vi "boonton_main.vi"() -> ()   [LabVIEW 2011]
uses:
  delay_time.vi
panel:
  out "Bias":string
  out "Loop Time 2":dbl
  in  "Sample Time":dbl
  out "Loop Time":dbl
  out "loop cnt":dbl
  in  "Destination File 2":path
  in  "Delay time":dbl
  in  "Destination File":path
  out "Command Read error out":errorcluster
  in  "Command File":path
  out "Result":string
  out "VISA error out":errorcluster
  in  "error in (no error)":errorcluster
  out "VISA Out":refnum<visa-resource-name>
  in  "VISA In":refnum<visa-resource-name>
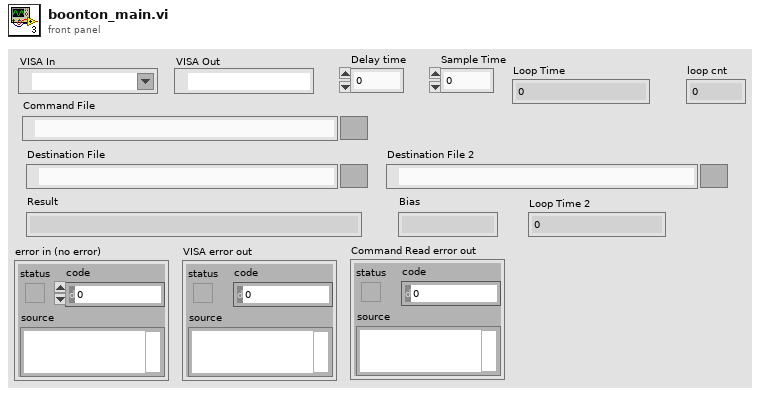
[diagram p1: front panel]
types:
  T1 = enum16{"open", "replace", "create", "open or create", "replace or create", "replace or create with confirmation"}
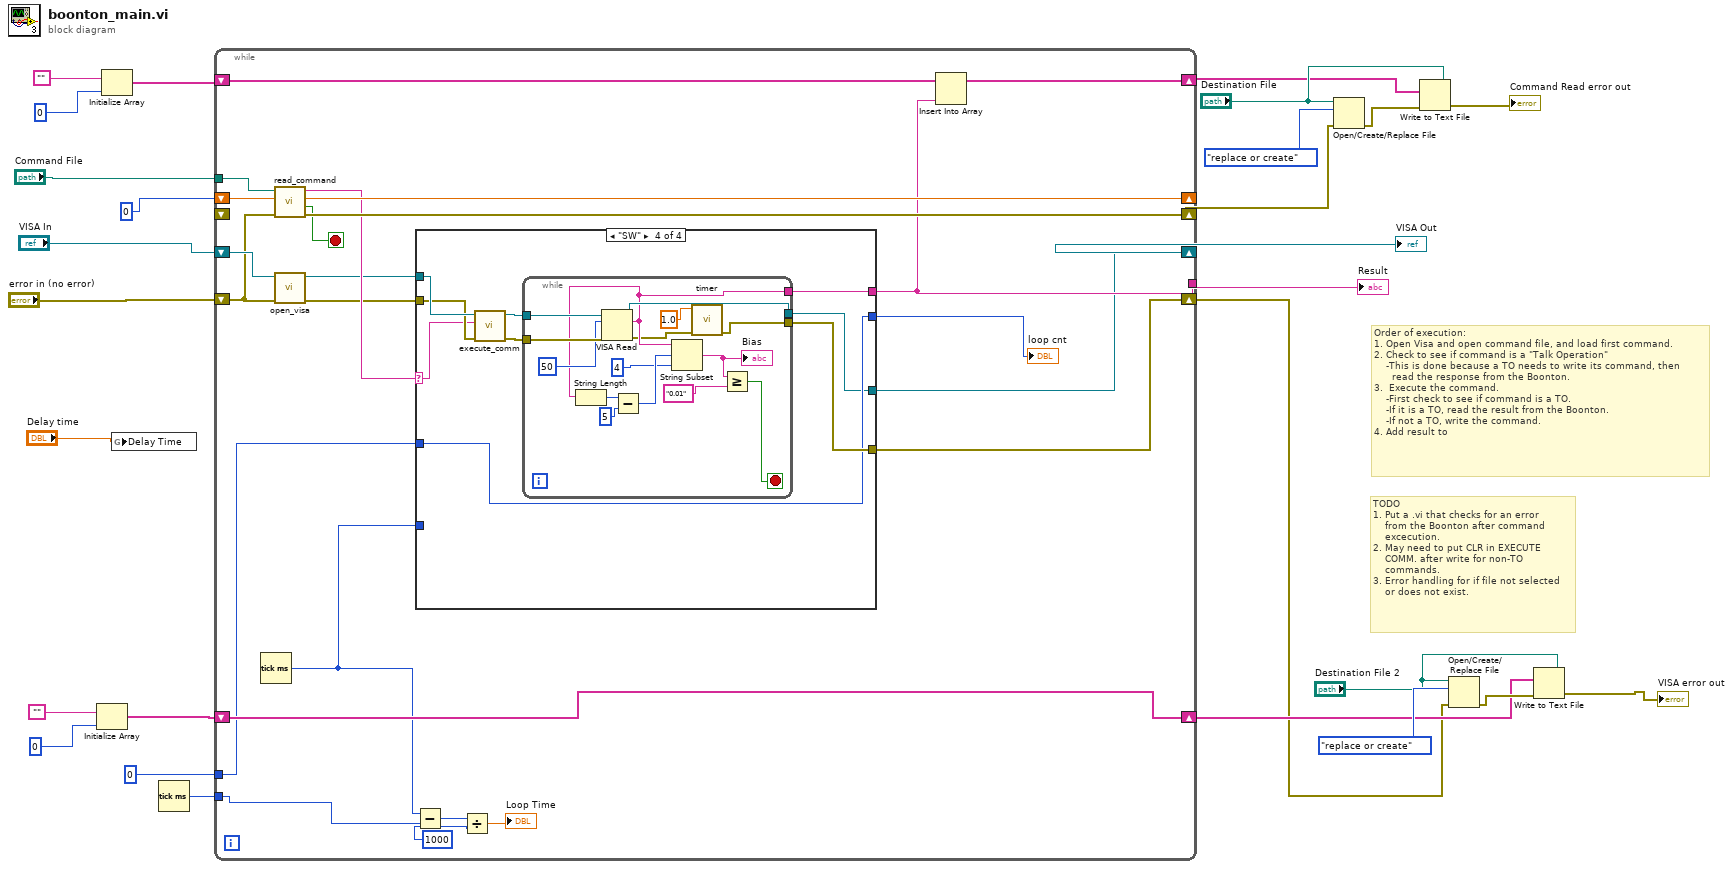
[diagram p0: block diagram]
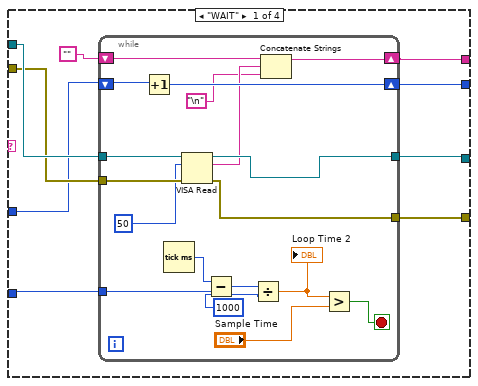
[diagram p2: hidden frame]
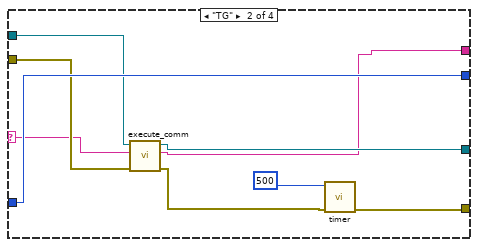
[diagram p3: hidden frame]
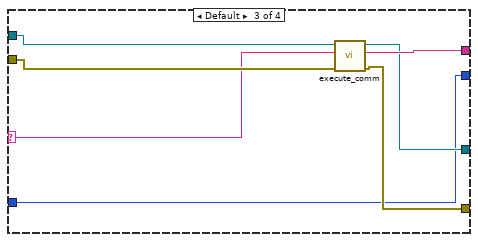
[diagram p4: hidden frame]
diagram:
  # "TODO\n1. Put a .vi that checks for an error\n    from the Boonton after command\n    excecution.\n2. May need to put CLR in EXECUTE\n    COMM. after write for non-TO\n    commands.\n3. Error handling for if file not selected\n    or does not exist."
  # "Order of execution:\n1. Open Visa and open command file, and load first command.\n2. Check to see if command is a \"Talk Operation\"\n    -This is done because a TO needs to write its command, then\n      read the response from the Boonton.\n3.  Execute the command.\n    -First check to see if command is a TO.\n    -If it is a TO, read the result from the Boonton.\n    -If not a TO, write the command.\n4. Add result to"
  n1 = Initialize Array("", 0) -> (w10:string[])
  n2 = Initialize Array("", 0) -> (w19:string[])
  n3 = global write "delay_time.vi" "Delay Time"("Delay time") -> ()
  n4 = Tick Count (ms)() -> (millisecond timer value=w3:u32)
  n5 = while {
    tunnel: [w36] -> w25
    tunnel: "Command File" -> [w47]
    shift-right: [w34] -> w26
    shift-left: "VISA In" -> [w50]
    shift-right: [w35] -> w4
    shift-left: "error in (no error)" -> [w49]
    shift-right: [w44] -> _
    shift-left: 0 -> [w46]
    shift-right: [w42] -> w15
    shift-left: w19 -> [w43]
    shift-right: [w48] -> w17
    shift-left: _ -> [_]
    shift-right: [w37] -> w6
    shift-left: w10 -> [w37]
    tunnel: w3 -> [w41]
    tunnel: 0 -> [w29]
    stop <- w45 stop-if-true
    n6 = Tick Count (ms)() -> (millisecond timer value=w30:u32)
    n7 = call "read_command.vi"("error in (no error)"=w49, "Current Comm. Num."=w46, "Path"=w47) -> ("error out"=w48:errorcluster, "Last Command  Reached"=w45:bool, "Next Comm. Num."=w44:dbl, "Command"=w33:string)  [unwired: 5 in]
    n8 = call "open_visa.vi"("error in (no error)"=w49, "VISA In"=w50) -> ("error out"=w31:errorcluster, "VISA Out"=w32:refnum<visa-resource-name>)  [unwired: 8 in]
    n9 = Subtract(x=w30, y=w41) -> (x-y=w39:u32)
    n10 = case shown="\"SW\"" w33 {
      selector: w33 -> [_ w81 w88 w100]
      tunnel: [w51 w78 w93 w95] -> w36
      tunnel: [w56 w85 w92 w97] -> w35
      tunnel: [w57 w79 w91 w94] -> w34
      tunnel: w32 -> [w59 w83 w90 w102]
      tunnel: w31 -> [w58 w82 w89 w101]
      tunnel: w30 -> [w55 _ _ _]
      tunnel: w29 -> [w54 w86 w87 w96]
      tunnel: [w53 w86 w87 w96] -> w28
      frame "WAIT" {
        n11 = while {
          tunnel: w59 -> [w77]
          tunnel: w58 -> [w76]
          tunnel: [w65] -> w57
          tunnel: [w64] -> w56
          tunnel: w55 -> [w72]
          shift-right: [w66] -> w53
          shift-left: w54 -> [w67]
          shift-right: [w61] -> w51
          shift-left: "" -> [w63]
          stop <- w71 stop-if-true
          n12 = Increment(x=w67) -> (x+1=w66:i32)
          n13 = Tick Count (ms)() -> (millisecond timer value=w75:u32)
          n14 = VISA Read(VISA resource name=w77, byte count=50, error in (no error)=w76) -> (VISA resource name out=w65:refnum<visa-resource-name>, read buffer=w62:string, error out=w64:errorcluster)  [unwired: 1 out]
          n15 = Subtract(x=w75, y=w72) -> (x-y=w74:u32)
          n16 = Divide(x=w74, y=1000) -> (x/y=w70:dbl)
          "Loop Time 2" <- w70
          n17 = Concatenate Strings(w63, w62, "\n") -> (w61:string)
          n18 = Greater?(x=w70, y="Sample Time") -> (0:w71:bool)
        }
      }
      frame "TG" {
        n19 = call "execute_comm.vi"("error in (no error)"=w82, "Command"=w81, "VISA In"=w83) -> ("error out"=w80:errorcluster, "Return Value"=w78:string, "VISA Out"=w79:refnum<visa-resource-name>)  [unwired: 6 in]
        n20 = call "timer.vi"("error in (no error)"=w80, "Delay Time"=500) -> ("error out"=w85:errorcluster)  [unwired: 9 in]
      }
      frame Default {
        n21 = call "execute_comm.vi"("error in (no error)"=w89, "Command"=w88, "VISA In"=w90) -> ("error out"=w92:errorcluster, "Return Value"=w93:string, "VISA Out"=w91:refnum<visa-resource-name>)  [unwired: 6 in]
      }
      frame "SW" {
        n22 = call "execute_comm.vi"("error in (no error)"=w101, "Command"=w100, "VISA In"=w102) -> ("error out"=w98:errorcluster, "VISA Out"=w99:refnum<visa-resource-name>)  [unwired: 6 in, 1 out]
        n23 = while {
          tunnel: w99 -> [w117]
          tunnel: w98 -> [w116]
          tunnel: [w115] -> w94
          tunnel: [w104] -> w97
          tunnel: [w109] -> w95
          stop <- w108 stop-if-true
          n24 = VISA Read(VISA resource name=w117, byte count=50, error in (no error)=w116) -> (VISA resource name out=w115:refnum<visa-resource-name>, read buffer=w109:string, error out=w105:errorcluster)  [unwired: 1 out]
          n25 = String Length(string=w109) -> (length=w113:i32)
          n26 = Subtract(x=w113, y=5) -> (x-y=w111:i32)
          n27 = String Subset(string=w109, offset (0)=w111, length (rest)=4) -> (substring=w107:string)
          "Bias" <- w107
          n28 = call "timer.vi"("error in (no error)"=w105, "Delay Time"=1.0) -> ("error out"=w104:errorcluster)  [unwired: 9 in]
          n29 = Greater Or Equal?(x=w107, y="0.01") -> (x >= y?=w108:bool)
        }
      }
    }
    "loop cnt" <- w28
    n30 = Divide(x=w39, y=1000) -> (x/y=→"Loop Time":dbl)
    n31 = Insert Into Array(array=w43, new element=w36) -> (w42:string[])  [unwired: 1 in]
  }
  "VISA Out" <- w26
  "Result" <- w25
  n32 = Open/Create/Replace File(file path (use dialog)="Destination File", error in=w17, operation (0:open)=T1."replace or create") -> (error out=w14:errorcluster)  [unwired: 3 in, 2 out]
  n33 = Write to Text File(file (use dialog)="Destination File", text=w15, error in=w14) -> (error out=→"Command Read error out":errorcluster)  [unwired: 1 in, 2 out]
  n34 = Open/Create/Replace File(file path (use dialog)="Destination File 2", error in=w4, operation (0:open)=T1."replace or create") -> (error out=w7:errorcluster)  [unwired: 3 in, 2 out]
  n35 = Write to Text File(file (use dialog)="Destination File 2", text=w6, error in=w7) -> (error out=→"VISA error out":errorcluster)  [unwired: 1 in, 2 out]
